vi "process_display.vi"(6 "error in (no error)":errorcluster) -> (0 "error out":errorcluster)   [LabVIEW 2010]
uses:
  typedefs/control_display_enum.ctl
  typedefs/data_cluster.ctl
panel:
  out "Ch2 (Stimulation)":waveform(dbl)(graph)
  out "Ch1 (Hamamatsu Avalanche Photodiode)":waveform(dbl)(graph)
  out "Ch0 (SensL Silicon Photomultiplier)":waveform(dbl)(graph)
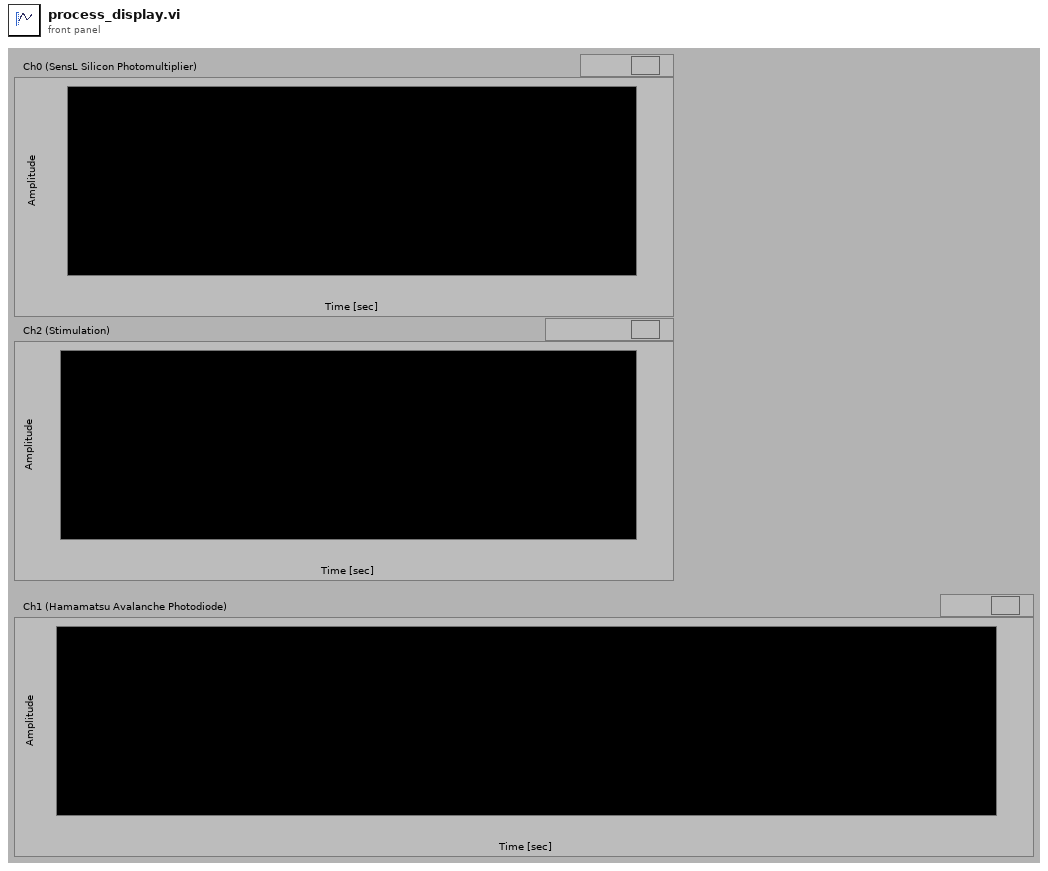
[diagram p1: front panel]
types:
  T1 = typedef "data_cluster.ctl" = cluster{"t0":dbl, "dt":dbl, "Channels":dbl[][]}
  T2 = typedef "control_display_enum.ctl" = enum16{"Init", "Display", "Quit"}
  T3 = cluster{"Control display enum":T2, "variant":variant}
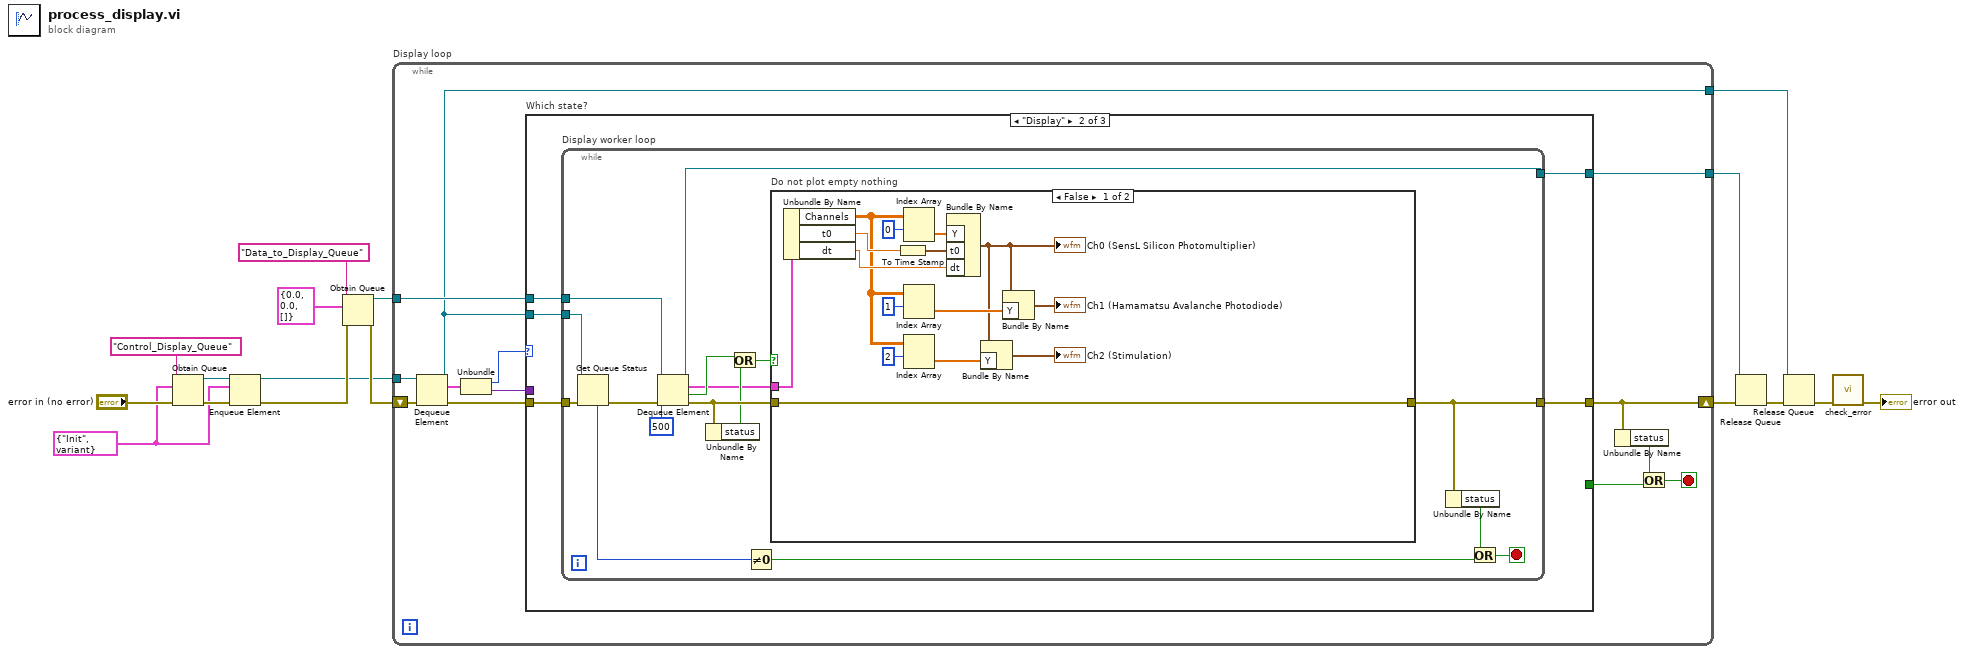
[diagram p0: block diagram]
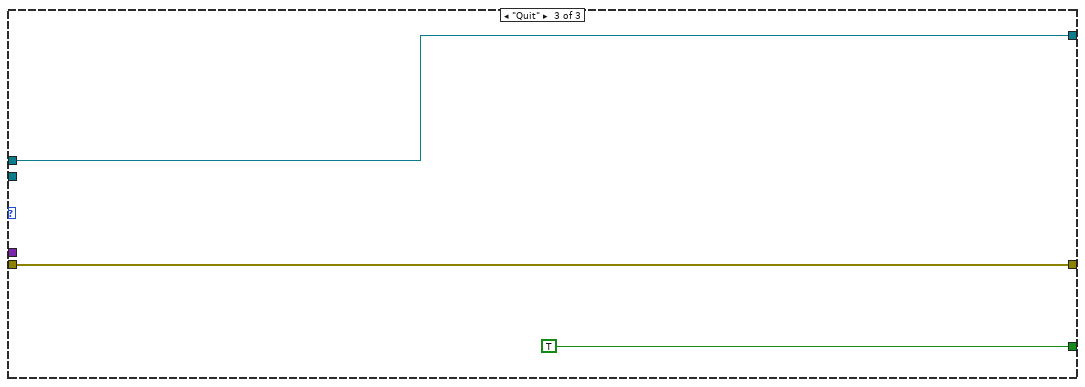
[diagram p4: hidden frame]
diagram:
  w9 = T3 {"Control display enum"=enum."Init", "variant"=variant}
  n1 = Obtain Queue(name (unnamed)="Control_Display_Queue", element data type=w9, error in (no error)="error in (no error)") -> (queue out=w8:refnum<queue>, error out=w11:errorcluster)  [unwired: 2 in, 1 out]
  n2 = Enqueue Element(queue=w8, element=w9, error in (no error)=w11) -> (queue out=w7:refnum<queue>, error out=w10:errorcluster)  [unwired: 1 in, 1 out]
  n3 = Obtain Queue(name (unnamed)="Data_to_Display_Queue", element data type=T1 {"t0"=0.0, "dt"=0.0, "Channels"=[]} ("Data cluster"), error in (no error)=w10) -> (queue out=w16:refnum<queue>, error out=w17:errorcluster)  [unwired: 2 in, 1 out]
  n4 = while "Display loop" {
    tunnel: w16 -> [w30]
    shift-right: [w29] -> w14
    shift-left: w17 -> [w28]
    tunnel: w7 -> [w26]
    tunnel: [w18] -> w4
    tunnel: [w22] -> w6
    stop <- w19 stop-if-true
    n5 = Dequeue Element(queue=w26, error in (no error)=w28) -> (queue out=w18:refnum<queue>, element=w25:T3, error out=w27:errorcluster)  [unwired: 1 in, 1 out]
    n6 = Unbundle(w25) -> ("Control display enum"=w24:T2, "variant"=w23:variant)
    n7 = case "Which state?" shown="\"Display\"" w24 {
      tunnel: w30 -> [w32 w37 w72]
      tunnel: w27 -> [w31 w36 w70]
      tunnel: [w31 w33 w70] -> w29
      tunnel: w23 -> [_ _ _]
      tunnel: [w32 w35 w72] -> w22
      tunnel: [_ _ TRUE] -> w21
      tunnel: w18 -> [_ w34 _]
      frame "Init", Default {
      }
      frame "Display" {
        n8 = while "Display worker loop" {
          tunnel: w37 -> [w53]
          tunnel: w36 -> [w47]
          tunnel: [w38] -> w33
          tunnel: [w52] -> w35
          tunnel: w34 -> [w44]
          stop <- w49 stop-if-true
          n9 = Get Queue Status(queue=w44, error in (no error)=w47) -> (error out=w46:errorcluster, # elements in queue=w51:i32)  [unwired: 1 in, 6 out]
          n10 = Dequeue Element(queue=w53, timeout in ms (-1)=500, error in (no error)=w46) -> (queue out=w52:refnum<queue>, element=w39:T1, timed out?=w40:bool, error out=w43:errorcluster)
          n11 = Unbundle By Name(w43) -> ("status"=w42:bool)
          n12 = Or(x=w40, y=w42) -> (x .or. y?=w41:bool)
          n13 = Not Equal To 0?(x=w51) -> (x != 0?=w48:bool)
          n14 = case "Do not plot empty nothing" shown="False" w41 {
            tunnel: [w54 w69] -> w38
            tunnel: w43 -> [w54 w69]
            tunnel: w39 -> [w68 _]
            frame False {
              n15 = Unbundle By Name(w68) -> ("Channels"=w60:dbl[][], "t0"=w64:dbl, "dt"=w63:dbl)
              n16 = To Time Stamp(1:w64) -> (0:w65:timestamp)
              n17 = Index Array(array=w60, index (row)=0) -> (element=w66:dbl[])  [unwired: 1 in]
              n18 = Index Array(array=w60, index (row)=1) -> (element=w61:dbl[])  [unwired: 1 in]
              n19 = Index Array(array=w60, index (row)=2) -> (element=w57:dbl[])  [unwired: 1 in]
              n20 = Bundle By Name("Y"=w66, "t0"=w65, "dt"=w63) -> (w56:waveform(dbl))  [unwired: 1 in]
              "Ch0 (SensL Silicon Photomultiplier)" <- w56
              n21 = Bundle By Name(cluster=w56, "Y"=w57) -> (→"Ch2 (Stimulation)":waveform(dbl))
              n22 = Bundle By Name(cluster=w56, "Y"=w61) -> (→"Ch1 (Hamamatsu Avalanche Photodiode)":waveform(dbl))
            }
            frame True {
            }
          }
          n23 = Unbundle By Name(w38) -> ("status"=w50:bool)
          n24 = Or(x=w50, y=w48) -> (x .or. y?=w49:bool)
        }
      }
      frame "Quit" {
      }
    }
    n25 = Unbundle By Name(w29) -> ("status"=w20:bool)
    n26 = Or(x=w20, y=w21) -> (x .or. y?=w19:bool)
  }
  n27 = Release Queue(queue=w6, error in (no error)=w14) -> (error out=w5:errorcluster)  [unwired: 1 in, 2 out]
  n28 = Release Queue(queue=w4, error in (no error)=w5) -> (error out=w2:errorcluster)  [unwired: 1 in, 2 out]
  n29 = call "check_error.vi"("error in"=w2) -> ("error out"=→"error out":errorcluster)  [unwired: 10 in]
